vi "Queue Nested Status.vi"(11 "Hello World Queue in":refnum<class "Hello World Queue.lvclass">) -> (0 "Queue Nested Count":i32, 1 "Queue Nested Aliases":string[](array[string]), 2 "Any Exist?":bool)   [LabVIEW 2021, in "Hello World Queue.lvlib" / "Hello World Queue.lvclass"]
uses:
  Hello World Queue.lvclass
  Hello World Queue.lvclass/Hello World Queue.ctl
  jettl/Queue jettl/Queue jettl.lvclass
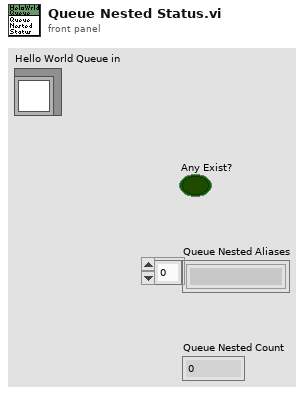
[diagram p1: front panel]
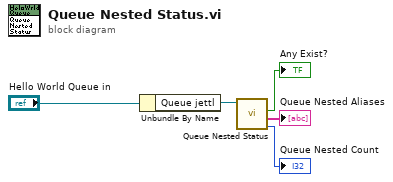
[diagram p0: block diagram]
diagram:
  n1 = Unbundle By Name("Hello World Queue in") -> ("Queue jettl"=w4:refnum<class "Queue jettl.lvclass">)
  n2 = call-dynamic "Queue Nested Status.vi"("jettl in"=w4) -> ("Queue Nested Count"=→"Queue Nested Count":i32, "Queue Nested Aliases"=→"Queue Nested Aliases":string[], "Any Exist?"=→"Any Exist?":bool)  [unwired: 8 in]
